vi "Is freestatement.vi"(1 "Variable Name":string) -> (0 "freestatement?":bool)   [LabVIEW 2019]
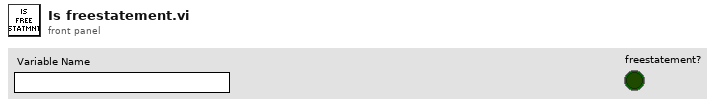
[diagram p1: front panel]
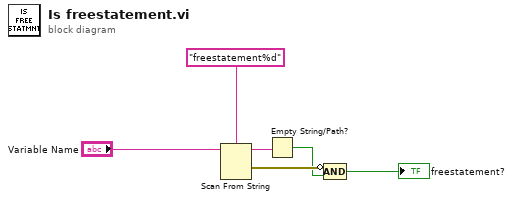
[diagram p0: block diagram]
diagram:
  n1 = Scan From String(format string="freestatement%d", input string="Variable Name") -> (remaining string=w3:string, error out=w4:errorcluster)  [unwired: 4 in, 1 out]
  n2 = Empty String/Path?(string/path=w3) -> (empty?=w2:bool)
  n3 = Compound Arithmetic op=AND(invert w4, w2) -> (→"freestatement?":bool)
